vi "PS90_PosVel.vi"(5 "read?":bool, 7 "Control unit ID":i32=1 min=1 max=10, 8 "error in (no error)":errorcluster, 9 "Value-In":i32 min=0, 10 "Axis number":i32=1 min=1 max=9, 11 "DLOwis.lvclass":refnum<class "DLOwis.lvclass">) -> (0 "error out":errorcluster, 1 "Value-Out":i32, 3 "DLOwis.lvclass":refnum<class "DLOwis.lvclass">)   [LabVIEW 2020, in "DLOwis.lvclass"]
doc: "PS90_PosVel.vi, created: 24.10.2006 alex; last change: 20.07.2016 alex;\n\n<B>FUNCTIONS:</B> \n\n<B>Read:</B> FALSE: read positioning velocity of an axis (internal values).\n<B>Write:</B> TRUE: set positioning velocity of an axis (internal values).\nIt is used for a trapezoidal and a S-curve profile.\n----------------------------------------------------------------------------------------\n<B>INPUT:</B>\n[TF] <B>function:</B> function selector. (Read, Write)\n[I32] <B>Control unit ID:</B> control unit index. (Default=1, Range=1...10)\n[I32] <B>Axis number:</B> axis number. (Default=1, Range=1...9)\n[I32] <B>Value-In:</B> velocity value. (only for Write: Default=0)\n[CLU] <B>error in</B>\n----------------------------------------------------------------------------------------\n<B>OUTPUT:</B>\n[I32] <B>Value-Out:</B> velocity value. (for Write: Value-Out=Value-In)\n[CLU] <B>error out</B>\n----------------------------------------------------------------------------------------\n<B>SUB-VIs:</B>\nPS90_GetReadError.vi\n----------------------------------------------------------------------------------------\n<B>EXT-Calls:</B>\nps90.dll (V2.00)\n----------------------------------------------------------------------------------------"
uses:
  DLOwis.lvclass
  C:/dev/TRANCON/Classes/Delay Line/DelayLine.lvclass
  DelayLine.lvclass/DelayLine.ctl
  DelayLine.lvclass
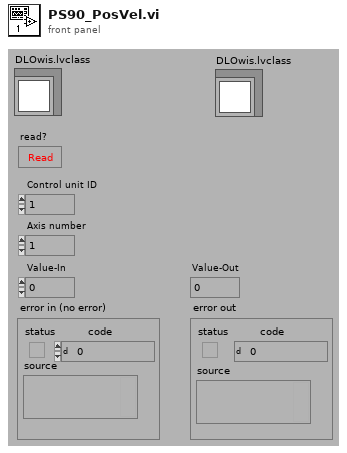
[diagram p1: front panel]
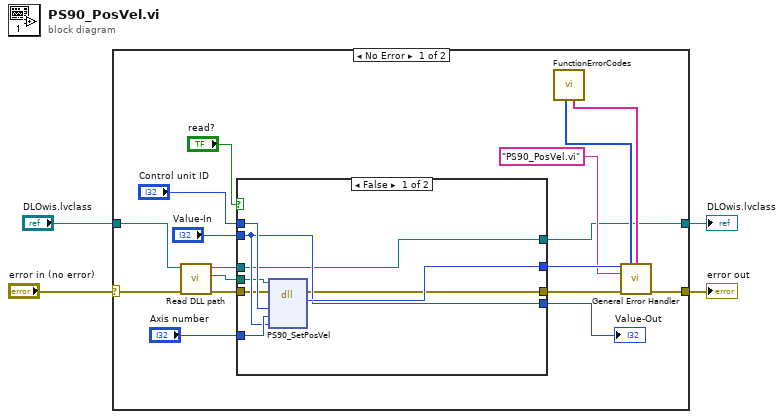
[diagram p0: block diagram]
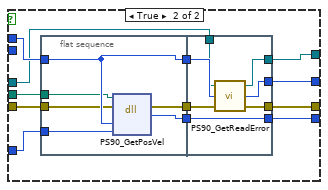
[diagram p2: hidden frame]
diagram:
  n1 = case shown="No Error" "error in (no error)" {
    selector: "error in (no error)" -> [w11 w55]
    tunnel: [w21 w55] -> w4
    tunnel: [w5 w56] -> w3
    tunnel: "DLOwis.lvclass" -> [w10 w56]
    frame No Error {
      n2 = call "Read DLL path.vi"("error in (no error)"=w11, "DelayLine in"=w10) -> ("error out"=w7:errorcluster, "DLL path"=w8:path, "DelayLine out"=w6:refnum<class "DLOwis.lvclass">)  [unwired: 7 in]
      n3 = case shown="False" "read?" {
        tunnel: "Control unit ID" -> [w28 w40]
        tunnel: [w29 w41] -> w18
        tunnel: "Value-In" -> [w26 _]
        tunnel: [w26 w39] -> w16
        tunnel: "Axis number" -> [w27 w38]
        tunnel: [w25 w31] -> w9
        tunnel: w8 -> [w22 w35]
        tunnel: w7 -> [w24 w34]
        tunnel: w6 -> [w23 w33]
        tunnel: [w23 w30] -> w5
        frame False {
          n4 = dll-call lib="C:/Users/Sergey Denisov/Documents/REPS/TRANCON/DLL/ps90.dll" fn="PS90_SetPosVel" label="PS90_Set\nPosVel"(path in=w22, error in=w24, "Index"=w28, "AxisNr"=w27, "Value"=w26) -> (error out=w25:errorcluster, "Rückgabetyp"=w29:i32)  [unwired: 4 in, 1 out]
        }
        frame True {
          n5 = flat-sequence {
            tunnel: w40 -> [w47]
            tunnel: [w47] -> w37
            tunnel: [w46] -> w36
            tunnel: w38 -> [w45]
            tunnel: w35 -> [w44]
            tunnel: w34 -> [w43]
            tunnel: [w42] -> w32
            tunnel: [w54] -> w41
            tunnel: w37 -> [w53]
            tunnel: [w52] -> w39
            tunnel: w36 -> [w52]
            tunnel: w33 -> [w51]
            tunnel: w32 -> [w50]
            tunnel: [w49] -> w31
            tunnel: [w48] -> w30
            frame #0 {
              n6 = dll-call lib="C:/Users/Sergey Denisov/Documents/REPS/TRANCON/DLL/ps90.dll" fn="PS90_GetPosVel" label="PS90_Get\nPosVel"(path in=w44, error in=w43, "Index"=w47, "AxisNr"=w45) -> (error out=w42:errorcluster, "Rückgabetyp"=w46:i32)  [unwired: 3 in, 1 out]
            }
            frame #1 {
              n7 = call "PS90_GetReadError.vi"("error in (no error)"=w50, "Control unit ID"=w53, "DLOwis.lvclass"=w51) -> ("error IO"=w49:errorcluster, "Read error"=w54:i32, "DLOwis.lvclass"=w48:refnum<class "DLOwis.lvclass">)
            }
          }
        }
      }
      "Value-Out" <- w16
      n8 = call "FunctionErrorCodes.vi"() -> ("[user-defined codes]"=w13:i32[], "[user-defined descriptions]"=w12:string[])  [unwired: 8 in]
      n9 = call <vilib>:"General Error Handler.vi"("[error code] (0)"=w18, "[user-defined codes]"=w13, "[user-defined descriptions]"=w12, "[error source] (\" \")"="PS90_PosVel.vi" ("[error source] (\" \")"), "error in (no error)"=w9) -> ("error out"=w21:errorcluster)  [unwired: 6 in, 4 out]
    }
    frame Error {
    }
  }
  "error out" <- w4
  "DLOwis.lvclass" <- w3
